vi "SW_Create_Images_overlay.vi"(3 "Blend factor":dbl=0.5 min=0.0 max=1.0, 4 "Background color":u32=16777216, 5 "Overlay Image":u32[][](array[numeric]), 6 "Background image":u32[][](array[numeric])) -> (1 "Conversion time, s":dbl, 2 "Output Image":u32[][](array[numeric]))   [LabVIEW 2018, in "Tracker.lvlib"]
uses:
  Tracker.lvlib
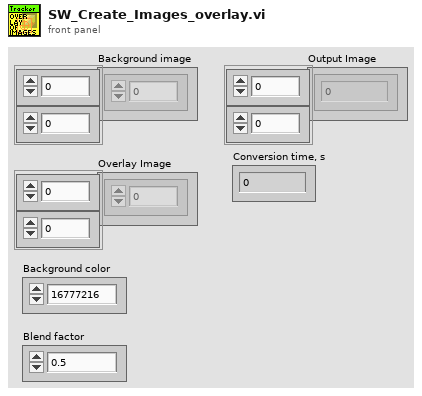
[diagram p1: front panel]
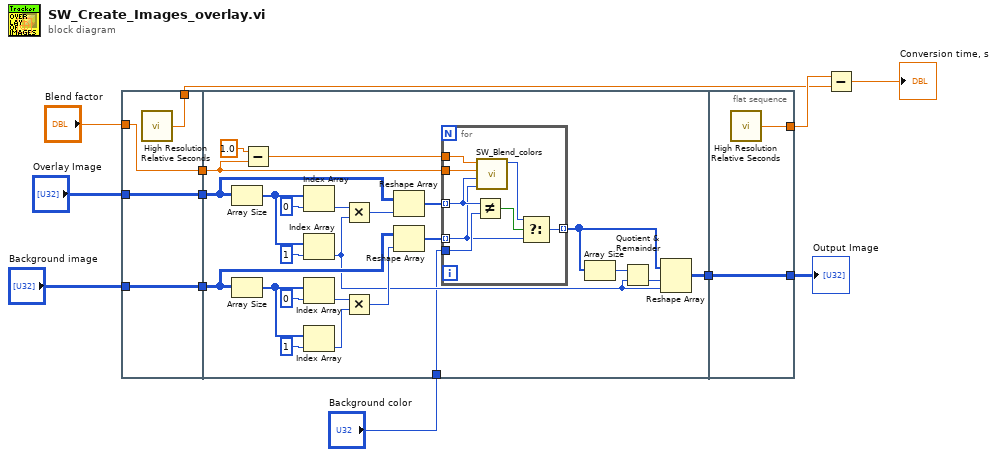
[diagram p0: block diagram]
diagram:
  n1 = flat-sequence {
    tunnel: "Background image" -> [w15]
    tunnel: "Overlay Image" -> [w16]
    tunnel: [w16] -> w9
    tunnel: [w15] -> w8
    tunnel: [w14] -> w5
    tunnel: [w13] -> w2
    tunnel: "Blend factor" -> [w13]
    tunnel: w9 -> [w40]
    tunnel: w8 -> [w39]
    tunnel: [w38] -> w7
    tunnel: "Background color" -> [w20]
    tunnel: w2 -> [w18]
    tunnel: [w50] -> w10
    tunnel: w7 -> [w50]
    tunnel: [w49] -> w6
    frame #0 {
      n2 = call <vilib>:"High Resolution Relative Seconds.vi"() -> ("relative seconds"=w14:dbl)
    }
    frame #1 {
      n3 = Array Size(array=w40) -> (size(s)=w27:i32[])
      n4 = Array Size(array=w39) -> (size(s)=w32:i32[])
      n5 = Subtract(x=1.0, y=w18) -> (x-y=w17:dbl)
      n6 = Index Array(array=w27, index=0) -> (element=w26:i32)
      n7 = Index Array(array=w27, index=1) -> (element=w21:i32)
      n8 = Index Array(array=w32, index=0) -> (element=w33:i32)
      n9 = Index Array(array=w32, index=1) -> (element=w35:i32)
      n10 = Multiply(x=w26, y=w21) -> (x*y=w25:i32)
      n11 = Multiply(x=w33, y=w35) -> (x*y=w34:i32)
      n12 = Reshape Array(w40, w25) -> (w37:u32[])
      n13 = Reshape Array(w39, w34) -> (w36:u32[])
      n14 = for {
        tunnel: w37 -> [w43] mode=indexing
        tunnel: w36 -> [w41] mode=indexing
        tunnel: [w48] -> w22 mode=indexing
        tunnel: w20 -> [w47]
        tunnel: w18 -> [w45]
        tunnel: w17 -> [w44]
        n15 = Not Equal?(x=w43, y=w47) -> (x != y?=w46:bool)
        n16 = call "SW_Blend_colors.vi"("Background color"=w41, "Overlay color"=w43, "Blend factor"=w45, "1 - Blend factor"=w44) -> ("Resulting color"=w42:u32)  [unwired: 7 in]
        n17 = Select(t=w42, s=w46, f=w41) -> (s? t:f=w48:u32)
      }
      n18 = Array Size(array=w22) -> (size(s)=w24:i32)
      n19 = Quotient & Remainder(x=w24, y=w21) -> (floor(x/y)=w23:i32)  [unwired: 1 out]
      n20 = Reshape Array(w22, w23, w21) -> (w38:u32[][])
    }
    frame #2 {
      n21 = call <vilib>:"High Resolution Relative Seconds.vi"() -> ("relative seconds"=w49:dbl)
    }
  }
  n22 = Subtract(x=w6, y=w5) -> (x-y=→"Conversion time, s":dbl)
  "Output Image" <- w10
